vi "CC FITS Calculate RA and DEC for Detector.vi"(8 "DEC":dbl, 9 "RA":dbl, 10 "ROT":dbl, 11 "Detector #":u16) -> (0 "error out":errorcluster, 1 "ROT out":dbl, 2 "DEC out":dbl, 3 "RA out":dbl)   [LabVIEW 2024]
panel:
  out "standard error":string
  in  "error in (no error)":errorcluster
  out "cmd prompt":string
  out "standard output":string
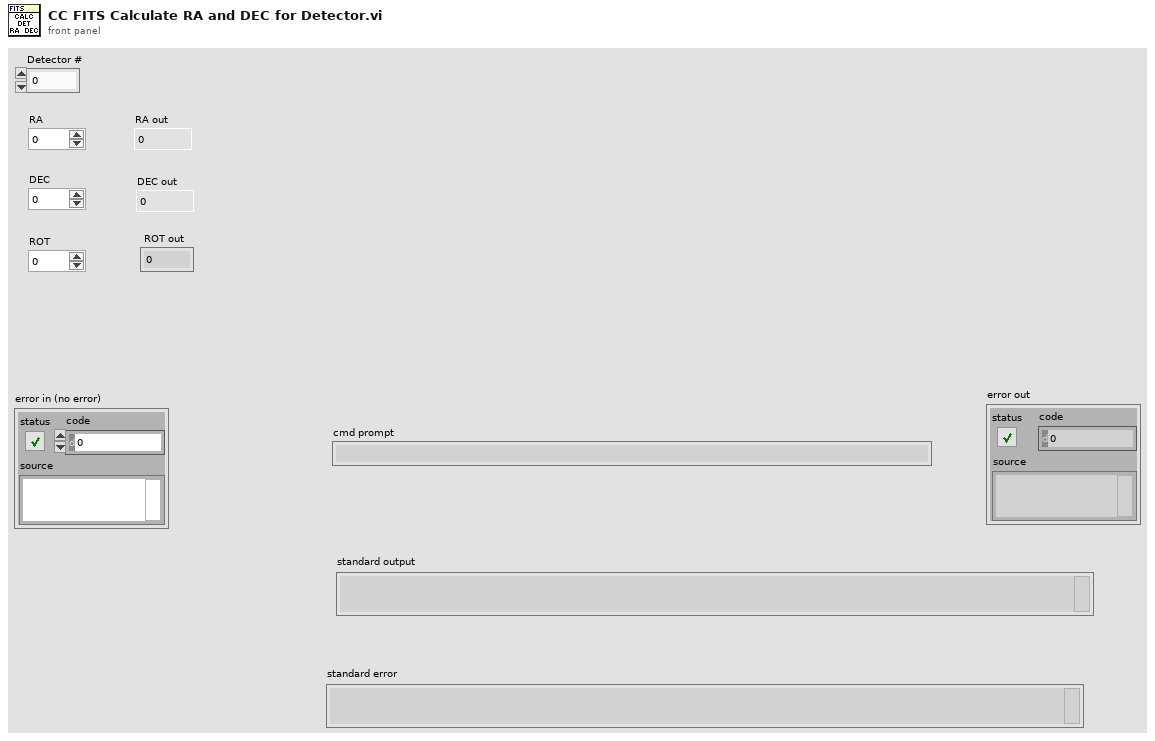
[diagram p1: front panel]
types:
  T1 = cluster{bool, "code":i32, "standard error":string}
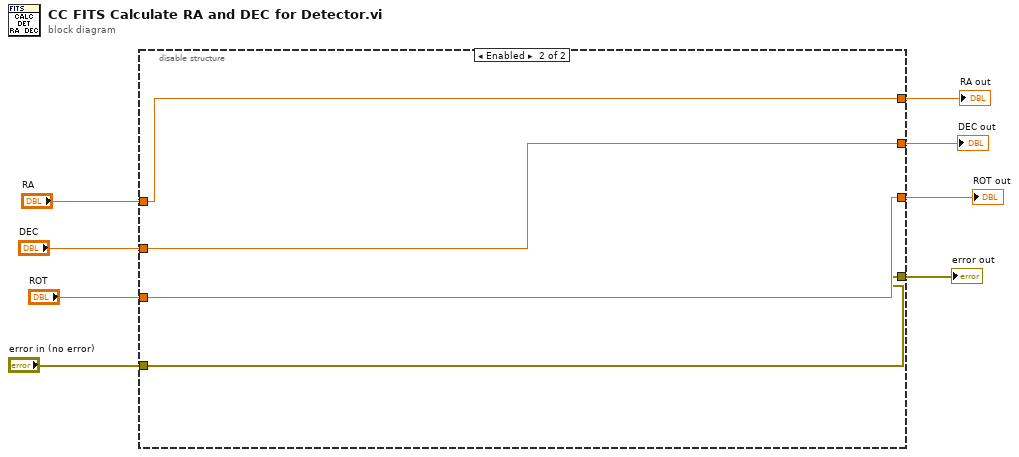
[diagram p0: block diagram]
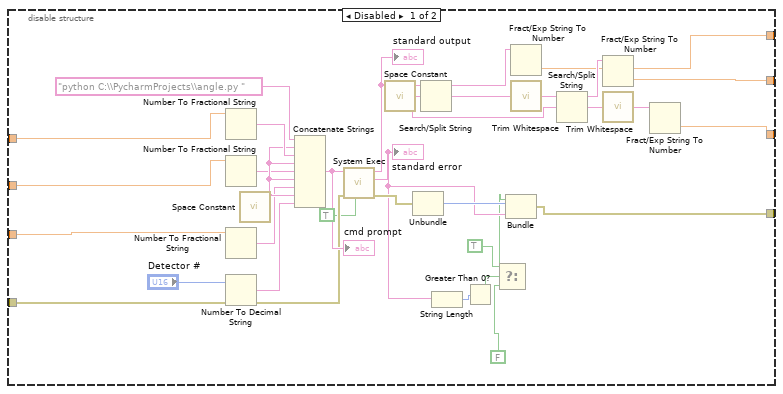
[diagram p2: hidden frame]
diagram:
  n1 = disable-structure shown="Enabled" {
    disable-tunnel: "ROT" -> [w38 w43]
    disable-tunnel: "DEC" -> [w37 w44]
    disable-tunnel: "RA" -> [w36 w45]
    disable-tunnel: "error in (no error)" -> [w29 w42]
    disable-tunnel: [w22 w45] -> w4
    disable-tunnel: [w21 w44] -> w3
    disable-tunnel: [w20 w43] -> w2
    disable-tunnel: [w9 w42] -> w1
    frame Disabled {
      n2 = Number To Fractional String(number=w36) -> (F-format string=w35:string)  [unwired: 3 in]
      n3 = Number To Fractional String(number=w37) -> (F-format string=w33:string)  [unwired: 3 in]
      n4 = Number To Fractional String(number=w38) -> (F-format string=w32:string)  [unwired: 3 in]
      n5 = Number To Decimal String(number="Detector #") -> (decimal integer string=w31:string)  [unwired: 1 in]
      n6 = call <vilib>:"Space Constant.vi"() -> ("String"=w34:string)
      n7 = Concatenate Strings("python C:\\PycharmProjects\\angle.py " ("command line"), w34, w35, w34, w33, w34, w32, w34, w31) -> (w41:string)
      "cmd prompt" <- w41
      n8 = call <vilib>:"System Exec.vi"("run minimized? (F)"=TRUE, "error in (no error)"=w29, "command line"=w41) -> ("error out"=w17:errorcluster, "standard error"=w15:string, "standard output"=w30:string)  [unwired: 5 in, 1 out]
      "standard output" <- w30
      "standard error" <- w15
      n9 = call <vilib>:"Space Constant.vi"() -> ("String"=w19:string)
      n10 = Unbundle(w17) -> ("code"=w16:i32)  [unwired: 2 out]
      n11 = Search/Split String(string=w30, search string/char (-)=w19) -> (substring before match=w28:string, match + rest of string=w27:string)  [unwired: 1 in, 1 out]
      n12 = String Length(string=w15) -> (length=w14:i32)
      n13 = Greater Than 0?(x=w14) -> (x > 0?=w13:bool)
      n14 = Select(t=TRUE, s=w13, f=FALSE) -> (s? t:f=w10:bool)
      n15 = Bundle(w10, "code"=w16, "standard error"=w15) -> (w9:T1)  [unwired: 1 in]
      n16 = Fract/Exp String To Number(string=w28) -> (number=w22:dbl)  [unwired: 3 in, 1 out]
      n17 = call <vilib>:"Trim Whitespace.vi"("string"=w27) -> ("trimmed string"=w26:string)  [unwired: 1 in]
      n18 = Search/Split String(string=w26, search string/char (-)=w19) -> (substring before match=w25:string, match + rest of string=w24:string)  [unwired: 1 in, 1 out]
      n19 = Fract/Exp String To Number(string=w25) -> (number=w21:dbl)  [unwired: 3 in, 1 out]
      n20 = call <vilib>:"Trim Whitespace.vi"("string"=w24) -> ("trimmed string"=w23:string)  [unwired: 1 in]
      n21 = Fract/Exp String To Number(string=w23) -> (number=w20:dbl)  [unwired: 3 in, 1 out]
    }
    frame Enabled {
    }
  }
  "DEC out" <- w3
  "RA out" <- w4
  "error out" <- w1
  "ROT out" <- w2
